vi "server.vi"() -> ()   [LabVIEW 2020]
panel:
  in  "stop":bool
  in  "Tamper":cluster{u32, u32}[](array[cluster])
  in  "Bypass":cluster{u32, u32}[](array[cluster])
  in  "Alarm":cluster{u32, u32}[](array[cluster])
  in  "Normal":cluster{u32, u32}[](array[cluster])
  out "Zone 1":bool
  # "Green : Normal\nRed : Alarm\nBlue : Bypass\nOrange: Tamper"
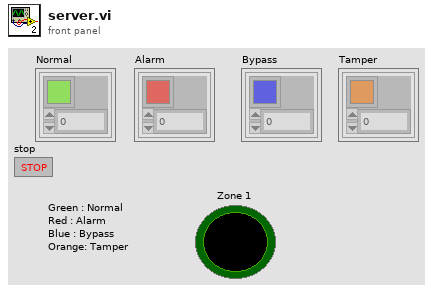
[diagram p1: front panel]
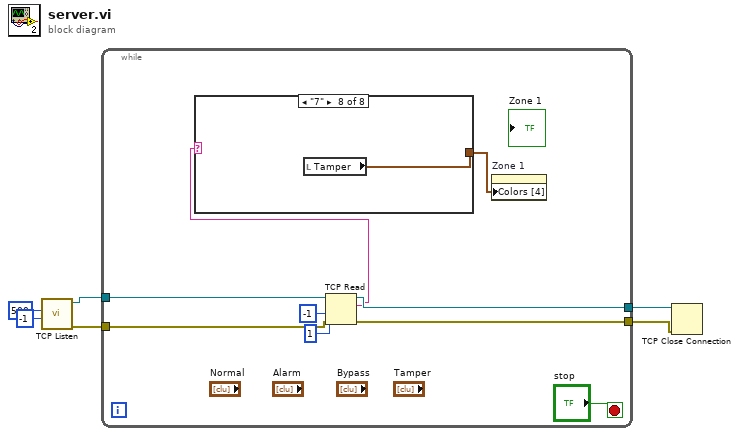
[diagram p0: block diagram]
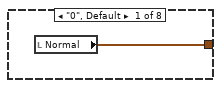
[diagram p2: hidden frame]
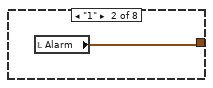
[diagram p3: hidden frame]
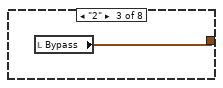
[diagram p4: hidden frame]
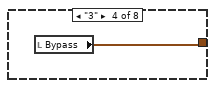
[diagram p5: hidden frame]
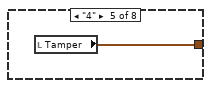
[diagram p6: hidden frame]
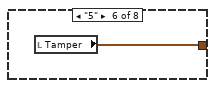
[diagram p7: hidden frame]
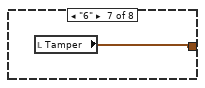
[diagram p8: hidden frame]
diagram:
  n1 = call <vilib>:"TCP Listen.vi"("timeout ms (wait forever: -1)"=-1, "port"=u16 500) -> ("error out"=w3:errorcluster, "connection ID"=w4:refnum<k5>)  [unwired: 5 in, 3 out]
  n2 = while {
    tunnel: w4 -> [w13]
    tunnel: w3 -> [w12]
    tunnel: [w11] -> w2
    tunnel: [w10] -> w1
    stop <- "stop" stop-if-true
    n3 = TCP Read(connection ID=w13, bytes to read=1, error in (no error)=w12, 9:-1 ("timeout ms (25000)")) -> (connection ID out=w11:refnum<k5>, data out=w9:string, error out=w10:errorcluster)  [unwired: 1 in]
    n4 = case shown="\"7\"" w9 {
      tunnel: [w16 w17 w18 w19 w20 w21 w22 w23] -> w8
      frame "0", Default {
        n5 = local read "Normal"() -> (w16:cluster{u32, u32}[])
      }
      frame "1" {
        n6 = local read "Alarm"() -> (w17:cluster{u32, u32}[])
      }
      frame "2" {
        n7 = local read "Bypass"() -> (w18:cluster{u32, u32}[])
      }
      frame "3" {
        n8 = local read "Bypass"() -> (w19:cluster{u32, u32}[])
      }
      frame "4" {
        n9 = local read "Tamper"() -> (w20:cluster{u32, u32}[])
      }
      frame "5" {
        n10 = local read "Tamper"() -> (w21:cluster{u32, u32}[])
      }
      frame "6" {
        n11 = local read "Tamper"() -> (w22:cluster{u32, u32}[])
      }
      frame "7" {
        n12 = local read "Tamper"() -> (w23:cluster{u32, u32}[])
      }
    }
    n13 = property on="Zone 1" class="Bool (strict)"("Colors [4]"=w8) -> ()  [unwired: 2 in, 2 out]
  }
  n14 = TCP Close Connection(connection ID=w2, error in (no error)=w1) -> ()  [unwired: 1 in, 2 out]
